vi "makeNewSVName.vi"(0 "HGF_DSCVarManager in":refnum<class "HGF_DSCVarManager.lvclass">, 2 "SV":string, 5 "error in (no error)":errorcluster) -> (14 "HGF_DSCVarManager out":refnum<class "HGF_DSCVarManager.lvclass">, 16 "SV out":string, 19 "error out":errorcluster)   [LabVIEW 2012, in "HGF_DSC.lvlib" / "HGF_DSCVarManager.lvclass"]
uses:
  HGF_DSCVarManager.lvclass
  HGF_DSCVarManager.lvclass/HGF_DSCVarManager.ctl
  <vilib>/lvdsc/NI_DSC.lvlib
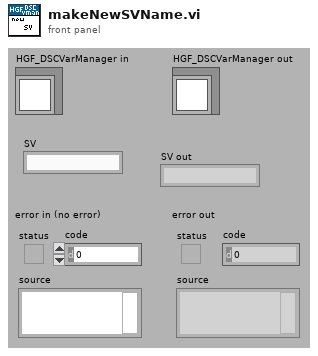
[diagram p1: front panel]
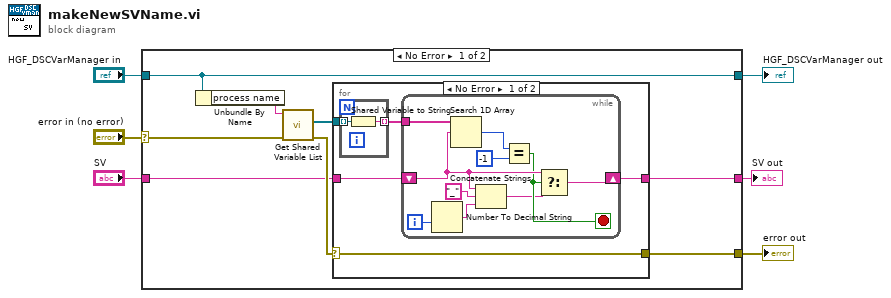
[diagram p0: block diagram]
diagram:
  n1 = case shown="No Error" "error in (no error)" {
    selector: "error in (no error)" -> [w7 w34]
    tunnel: [w10 w34] -> w5
    tunnel: [w8 w33] -> w3
    tunnel: "HGF_DSCVarManager in" -> [w8 w33]
    tunnel: "SV" -> [w12 _]
    tunnel: [w11 _] -> w1
    frame No Error {
      n2 = Unbundle By Name(w8) -> ("process name"=w9:string)
      n3 = call <vilib>:"Get Shared Variable List.vi"("error in (no error)"=w7, "process name"=w9) -> ("error out"=w14:errorcluster, "shared variables"=w13:refnum<k21>[])  [unwired: 8 out]
      n4 = case shown="No Error" w14 {
        selector: w14 -> [w15 w32]
        tunnel: w13 -> [w19 _]
        tunnel: w12 -> [w17 _]
        tunnel: [w16 _] -> w11
        tunnel: [w15 w32] -> w10
        frame No Error {
          n5 = for {
            tunnel: w19 -> [w31] mode=indexing
            tunnel: [w30] -> w18 mode=indexing
            n6 = Shared Variable to String(1:w31) -> (0:w30:string)
          }
          n7 = while {
            tunnel: w18 -> [w29]
            shift-right: [w26] -> w16
            shift-left: w17 -> [w25]
            i -> [w23]
            stop <- w21 stop-if-true
            n8 = Number To Decimal String(number=w23) -> (decimal integer string=w22:string)  [unwired: 1 out]
            n9 = Search 1D Array(1D array=w29, element=w25) -> (index of element=w28:i32)  [unwired: 1 out]
            n10 = Concatenate Strings(w25, "_" ("string"), w22) -> (w20:string)
            n11 = Equal?(x=w28, y=-1) -> (x = y?=w21:bool)
            n12 = Select(t=w25, s=w21, f=w20) -> (s? t:f=w26:string)
          }
        }
        frame Error {
        }
      }
    }
    frame Error {
    }
  }
  "error out" <- w5
  "HGF_DSCVarManager out" <- w3
  "SV out" <- w1
